vi "Generate 1D Motion Profile.vi"(0 "Target Position":dbl, 1 "Initial Velocity (0)":dbl format="%#_13g", 3 "Final Velocity (0)":dbl format="%#_13g", 5 "Initial Position (0)":dbl format="%#_13g", 7 "Max Velocity":dbl, 9 "Max Acceleration":dbl, 11 "Error In":errorcluster, 12 "resolution m (.001)":dbl=0.001 format="%#_13g") -> (4 "Time Plot":T1, 6 "Distance vs Velocity":cluster{"Position":dbl[], "Velocity":dbl[]}, 15 "Error Out":errorcluster)   [LabVIEW 2015]
uses:
  <vilib>/Analysis/NI_AALPro.lvlib
panel:
  out "Distance vs Velocity":cluster{dbl[], dbl[]}(graph)
  out "Perfect Path":cluster{"Integral X":dbl[], dbl[]}[](graph)
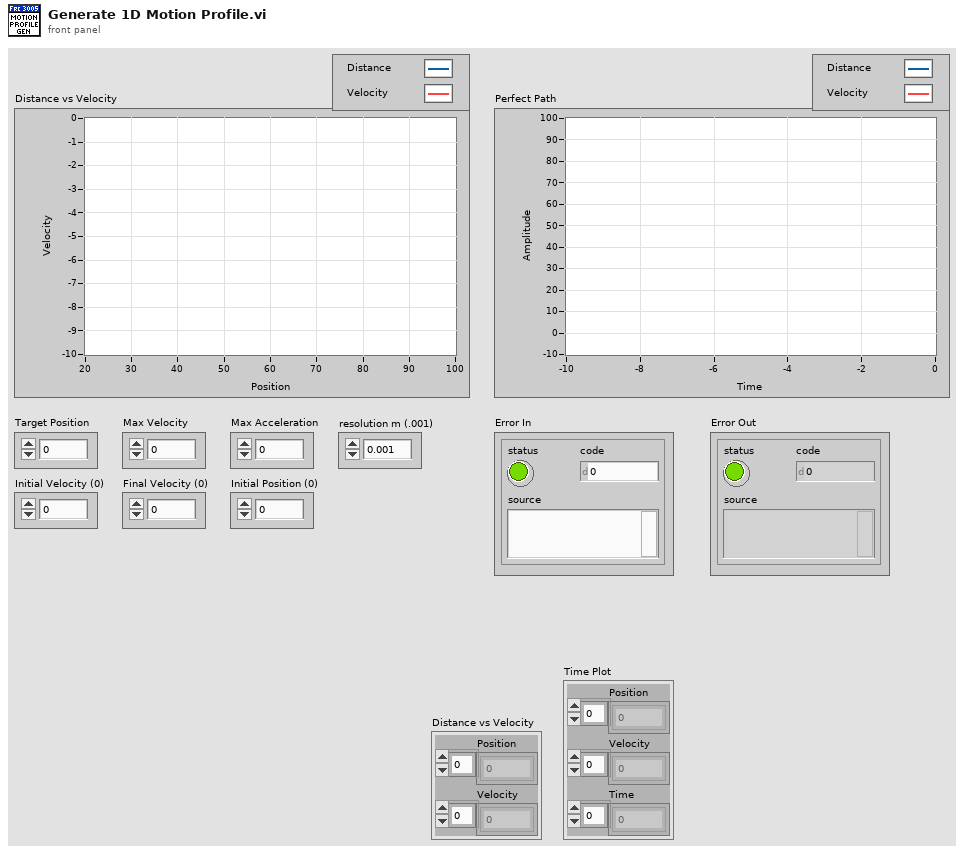
[diagram p1: front panel]
types:
  T1 = cluster{"Position":dbl[], "Velocity":dbl[], "Time":dbl[]}
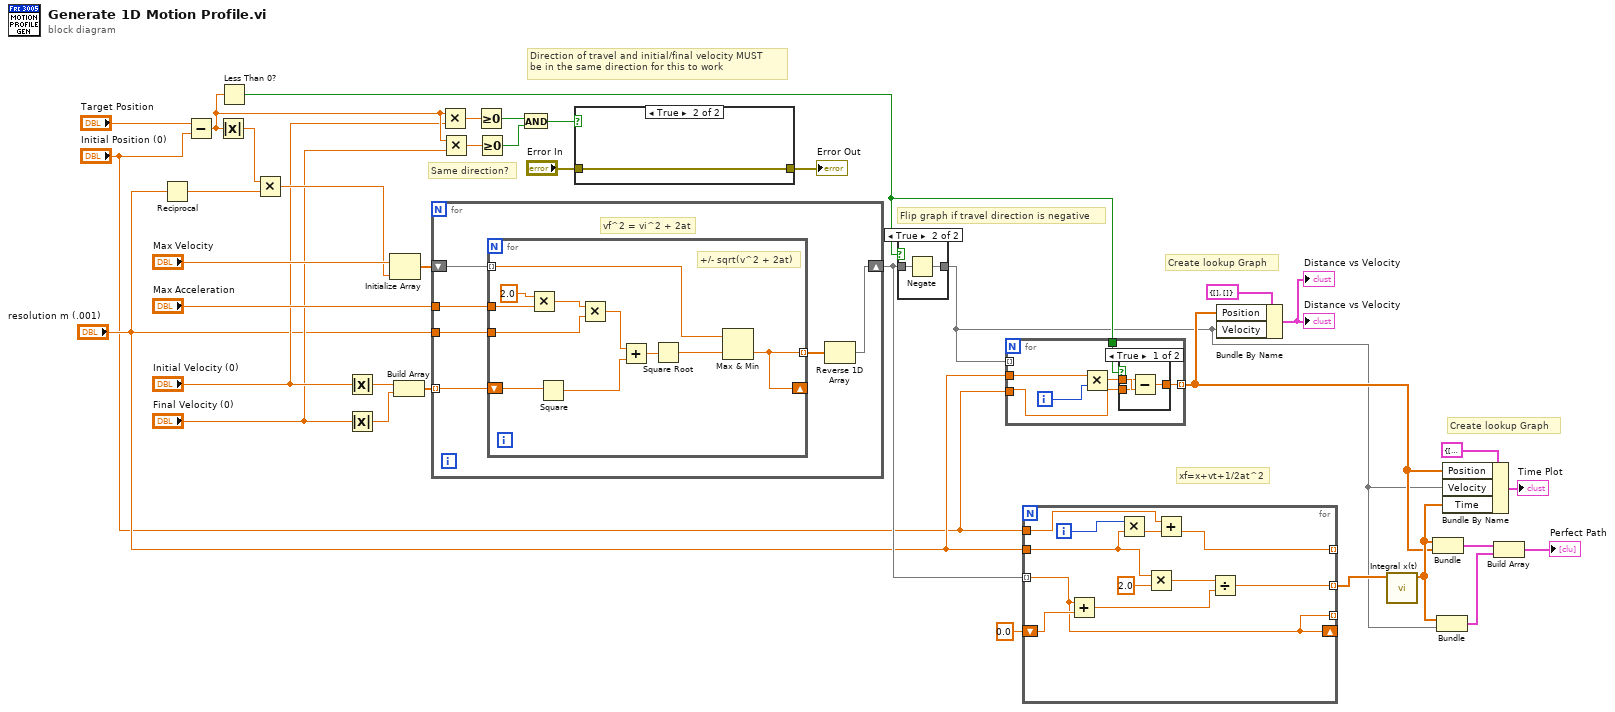
[diagram p0: block diagram]
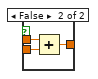
[diagram p2: hidden frame]
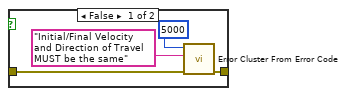
[diagram p3: hidden frame]
diagram:
  # "Create lookup Graph"
  # "Create lookup Graph"
  # "Same direction?"
  # "Flip graph if travel direction is negative"
  # "Direction of travel and initial/final velocity MUST\nbe in the same direction for this to work"
  # "xf=x+vt+1/2at^2"
  n1 = Reciprocal(x="resolution m (.001)") -> (1/x=w36:dbl)
  n2 = Subtract(x="Target Position", y="Initial Position (0)") -> (x-y=w18:dbl)
  n3 = Absolute Value(x=w18) -> (abs(x)=w30:dbl)
  n4 = Less Than 0?(x=w18) -> (x < 0?=w14:bool)
  n5 = Multiply(x=w30, y=w36) -> (x*y=w32:dbl)
  n6 = Absolute Value(x="Initial Velocity (0)") -> (abs(x)=w27:dbl)
  n7 = Absolute Value(x="Final Velocity (0)") -> (abs(x)=w28:dbl)
  n8 = Initialize Array("Max Velocity", w32) -> (w33:dbl[])
  n9 = Build Array(w27, w28) -> (w29:dbl[])
  n10 = for {
    tunnel: "Max Acceleration" -> [w41]
    tunnel: w29 -> [w38] mode=indexing
    tunnel: "resolution m (.001)" -> [w40]
    shift-right: [w42] -> w26
    shift-left: w33 -> [w39]
    # "vf^2 = vi^2 + 2at"
    n11 = for {
      shift-right: [w52] -> _
      shift-left: w38 -> [w44]
      tunnel: [w52] -> w37 mode=indexing
      tunnel: w41 -> [w50]
      tunnel: w39 -> [w53] mode=indexing
      tunnel: w40 -> [w51]
      # "+/- sqrt(v^2 + 2at)"
      n12 = Multiply(x=2.0, y=w50) -> (x*y=w49:dbl)
      n13 = Square(x=w44) -> (x^2=w46:dbl)
      n14 = Multiply(x=w49, y=w51) -> (x*y=w47:dbl)
      n15 = Add(x=w47, y=w46) -> (x+y=w45:dbl)
      n16 = Square Root(x=w45) -> (sqrt(x)=w43:dbl)
      n17 = Max & Min(x=w53, y=w43) -> (min(x,y)=w52:dbl)  [unwired: 1 out]
    }
    n18 = Reverse 1D Array(array=w37) -> (reversed array=w42:dbl[])
  }
  n19 = Multiply(x=w18, y="Initial Velocity (0)") -> (x*y=w20:dbl)
  n20 = Multiply(x=w18, y="Final Velocity (0)") -> (x*y=w21:dbl)
  n21 = Greater Or Equal To 0?(x=w20) -> (x >= 0?=w23:bool)
  n22 = Greater Or Equal To 0?(x=w21) -> (x >= 0?=w19:bool)
  n23 = And(x=w23, y=w19) -> (x .and. y?=w22:bool)
  n24 = case shown="True" w22 {
    tunnel: [w55 w58] -> w25
    tunnel: "Error In" -> [w54 w58]
    frame False {
      n25 = call <vilib>:"Error Cluster From Error Code.vi"("error in (no error)"=w54, "error message (\"\")"="Initial/Final Velocity and Direction of Travel MUST be the same" ("error message (\"\")"), "error code (0)"=5000) -> ("error out"=w55:errorcluster)  [unwired: 6 in]
    }
    frame True {
    }
  }
  "Error Out" <- w25
  n26 = case shown="True" w14 {
    tunnel: w26 -> [w59 w61]
    tunnel: [w59 w60] -> w1
    frame False {
    }
    frame True {
      n27 = Negate(x=w61) -> (-x=w60:dbl[])
    }
  }
  n28 = for {
    tunnel: "resolution m (.001)" -> [w67]
    tunnel: "Initial Position (0)" -> [w64]
    tunnel: [w63] -> w2 mode=indexing
    tunnel: w1 -> [_] mode=indexing
    tunnel: w14 -> [w62]
    i -> [w66]
    n29 = Multiply(x=w67, y=w66) -> (x*y=w65:dbl)
    n30 = case shown="True" w62 {
      tunnel: w65 -> [w70 w73]
      tunnel: w64 -> [w69 w72]
      tunnel: [w68 w71] -> w63
      frame True {
        n31 = Subtract(x=w69, y=w70) -> (x-y=w68:dbl)
      }
      frame False {
        n32 = Add(x=w73, y=w72) -> (x+y=w71:dbl)
      }
    }
  }
  n33 = for {
    tunnel: w26 -> [w80] mode=indexing
    shift-right: [w80] -> _
    shift-left: 0.0 ("Max Velocity") -> [w82]
    tunnel: "resolution m (.001)" -> [w76]
    tunnel: [w75] -> _ mode=indexing
    tunnel: [w80] -> _ mode=indexing
    tunnel: [w78] -> w11 mode=indexing
    tunnel: "Initial Position (0)" -> [w74]
    i -> [w79]
    n34 = Add(x=w80, y=w82) -> (x+y=w81:dbl)
    n35 = Multiply(x=w79, y=w76) -> (x*y=w77:dbl)
    n36 = Multiply(x=w76, y=2.0) -> (x*y=w83:dbl)
    n37 = Add(x=w74, y=w77) -> (x+y=w75:dbl)
    n38 = Divide(x=w83, y=w81) -> (x/y=w78:dbl)
  }
  n39 = Bundle By Name(cluster=cluster{"Position":dbl[], "Velocity":dbl[]} {"Position"=[], "Velocity"=[]}, "Position"=w2, "Velocity"=w1) -> (→"Distance vs Velocity" →"Distance vs Velocity":cluster{"Position":dbl[], "Velocity":dbl[]})
  n40 = call <vilib>:"Integral x(t).vi"("X"=w11) -> ("Integral X"=w5:dbl[])  [unwired: 9 in, 1 out]
  n41 = Bundle("Integral X"=w5, w2) -> (w9:cluster{"Integral X":dbl[], dbl[]})  [unwired: 1 in]
  n42 = Bundle("Integral X"=w5, w1) -> (w10:cluster{"Integral X":dbl[], dbl[]})  [unwired: 1 in]
  n43 = Bundle By Name(cluster=T1 {"Position"=[], "Velocity"=[], "Time"=[]}, "Position"=w2, "Velocity"=w1, "Time"=w5) -> (→"Time Plot":T1)
  n44 = Build Array(w9, w10) -> (→"Perfect Path":cluster{"Integral X":dbl[], dbl[]}[])
